vi "Direttore.fpga.vi"   [LabVIEW 2012]
uses:
  <vilib>/rvi/interface/RandomDataEmulation/nirviRandomDataFPGAFIFO.vi
  <vilib>/rvi/interface/RandomDataEmulation/niFpgaRandomDataHandleErrors.vi
  <vilib>/rvi/DataTransferAndStorage/Container/XNode/niFpgaContainer.xnode
  <vilib>/rvi/interface/RandomDataEmulation/nirviRandomDataFpgaReadWriteTemplate.vi
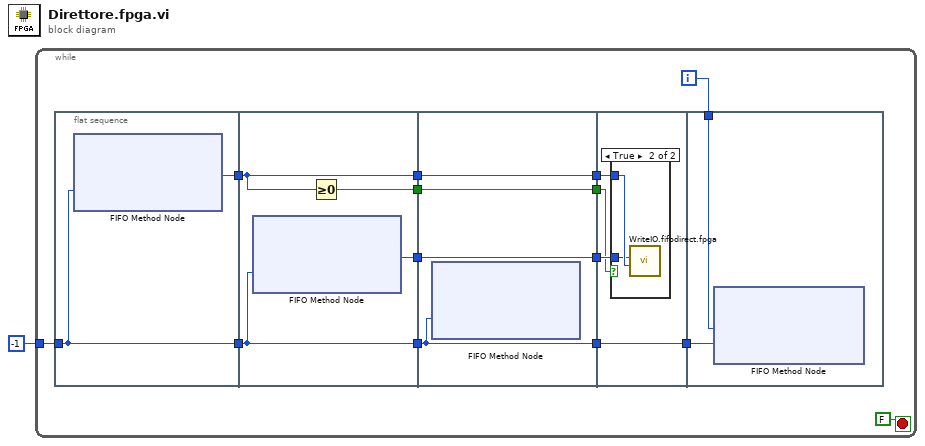
[diagram p0: block diagram]
diagram:
  n1 = while {
    tunnel: -1 ("Timeout") -> [w13]
    i -> [w2]
    stop <- FALSE stop-if-true
    n2 = flat-sequence {
      tunnel: w13 -> [w17]
      tunnel: [w17] -> w11
      tunnel: [w16] -> w9
      tunnel: [w20] -> w12
      tunnel: w11 -> [w21]
      tunnel: [w21] -> w10
      tunnel: w9 -> [w18]
      tunnel: [w18] -> w8
      tunnel: [w19] -> w7
      tunnel: [w23] -> w15
      tunnel: [w25] -> w14
      tunnel: w12 -> [w23]
      tunnel: w10 -> [w22]
      tunnel: w8 -> [w25]
      tunnel: w7 -> [w24]
      tunnel: [w24] -> w6
      tunnel: [w22] -> w4
      tunnel: w15 -> [w28]
      tunnel: w14 -> [w29]
      tunnel: w6 -> [w27]
      tunnel: w4 -> [w26]
      tunnel: [w26] -> w3
      tunnel: w3 -> [w33]
      tunnel: w2 -> [w32]
      frame #0 {
        n3 = xnode ("FIFO Method Node")("Timeout"=w17) -> ("Element"=w16:i32)  [unwired: 1 in, 2 out]
      }
      frame #1 {
        n4 = xnode ("FIFO Method Node")("Timeout"=w21) -> ("Element"=w20:i32)  [unwired: 1 in, 2 out]
        n5 = Greater Or Equal To 0?(x=w18) -> (x >= 0?=w19:bool)
      }
      frame #2 {
        n6 = xnode ("FIFO Method Node")("Timeout"=w22) -> ()  [unwired: 1 in, 3 out]
      }
      frame #3 {
        n7 = case shown="True" w27 {
          tunnel: w28 -> [_ w30]
          tunnel: w29 -> [_ w31]
          frame False {
          }
          frame True {
            n8 = call "WriteIO.fifodirect.fpga.vi"("Delta time"=w31, "Number of time points"=w30) -> ()  [unwired: 10 in]
          }
        }
      }
      frame #4 {
        n9 = xnode ("FIFO Method Node")("Element"=w32, "Timeout"=w33) -> ()  [unwired: 1 in, 2 out]
      }
    }
  }
